vi "Circulo.vi"() -> ()   [LabVIEW 2020]
panel:
  out "Grafico de un Circulo":cluster{dbl[], dbl[]}(graph)
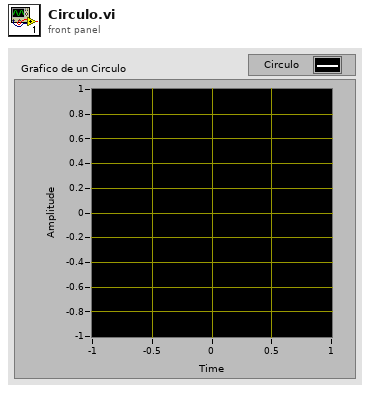
[diagram p1: front panel]
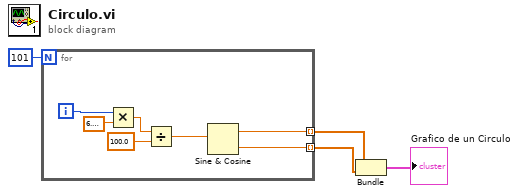
[diagram p0: block diagram]
diagram:
  n1 = for {
    N: 101 -> [_]
    tunnel: [w10] -> w4 mode=indexing
    tunnel: [w9] -> w3 mode=indexing
    i -> [w6]
    n2 = Multiply(x=w6, y=6.283185307179586) -> (x*y=w11:dbl)
    n3 = Divide(x=w11, y=100.0) -> (x/y=w5:dbl)
    n4 = Sine & Cosine(0:w5) -> (1:w10:dbl, 2:w9:dbl)
  }
  n5 = Bundle(w4, w3) -> (→"Grafico de un Circulo":cluster{dbl[], dbl[]})  [unwired: 1 in]
